vi "coord 2 bound.vi"(10 "Target Size (px)":dbl, 11 "Coordinates":dbl[](array[numeric])) -> (3 "bound":cluster{sgl, sgl, sgl, sgl})   [LabVIEW 2019]
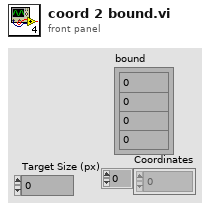
[diagram p1: front panel]
types:
  T1 = cluster{"Left":i32, "Top":i32, "Right":i32, "Bottom":i32}
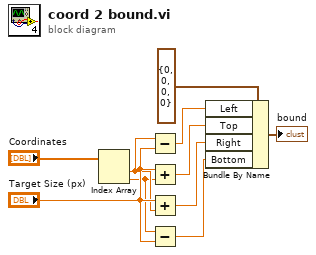
[diagram p0: block diagram]
diagram:
  n1 = Index Array(array="Coordinates") -> (element #1=w2:dbl, element #2=w1:dbl)  [unwired: 2 in]
  n2 = Subtract(x=w2, y="Target Size (px)") -> (x-y=w5:dbl)
  n3 = Add(x="Target Size (px)", y=w1) -> (x+y=w7:dbl)
  n4 = Add(x="Target Size (px)", y=w2) -> (x+y=w6:dbl)
  n5 = Subtract(x=w1, y="Target Size (px)") -> (x-y=w8:dbl)
  n6 = Bundle By Name(cluster=T1 {"Left"=0, "Top"=0, "Right"=0, "Bottom"=0} ("Bounding Rectangle"), "Left"=w5, "Top"=w7, "Right"=w6, "Bottom"=w8) -> (→"bound":T1)
